vi "Test Plan - New Template (SubVI).vi"(8 "error in":errorcluster, 11 "Test Plan Name":string) -> (0 "error out":errorcluster, 2 "Give a name for new Test Plan 2":string, 3 "Test Type 2":T1 items=["Please Select", "Triaxial Shear", "Triaxial UU", "Shearbox", "Permeability", "Consolidation (Stepped Loading)/Swelling", "Saturation (Incremental)", "User Defined", "UCT", "Isotropic Consolidation"], 5 "save?":bool)   [LabVIEW 2019]
uses:
  Controls/Station - Test Type.ctl
  Controls/Test plan select-state.ctl
panel:
  in  "Test Type":u16(ring) items=["Please Select", "Triaxial Shear", "Triaxial UU", "Shearbox", "Permeability", "Consolidation (Stepped Loading)/Swelling", "Saturation (Incremental)", "User Defined", "UCT", "Isotropic Consolidation"]
  in  "OK":bool
  in  "Cancel":bool
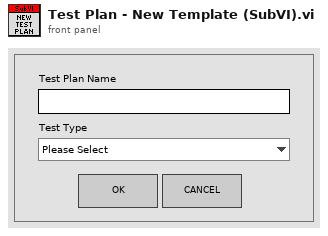
[diagram p1: front panel]
types:
  T1 = typedef "Station - Test Type.ctl" = u16
  T2 = enum16{"open", "replace", "create", "open or create", "replace or create", "replace or create with confirmation"}
  T3 = typedef "Test plan select-state.ctl" = enum16{"Init", "Idle", "Save", "Close"}
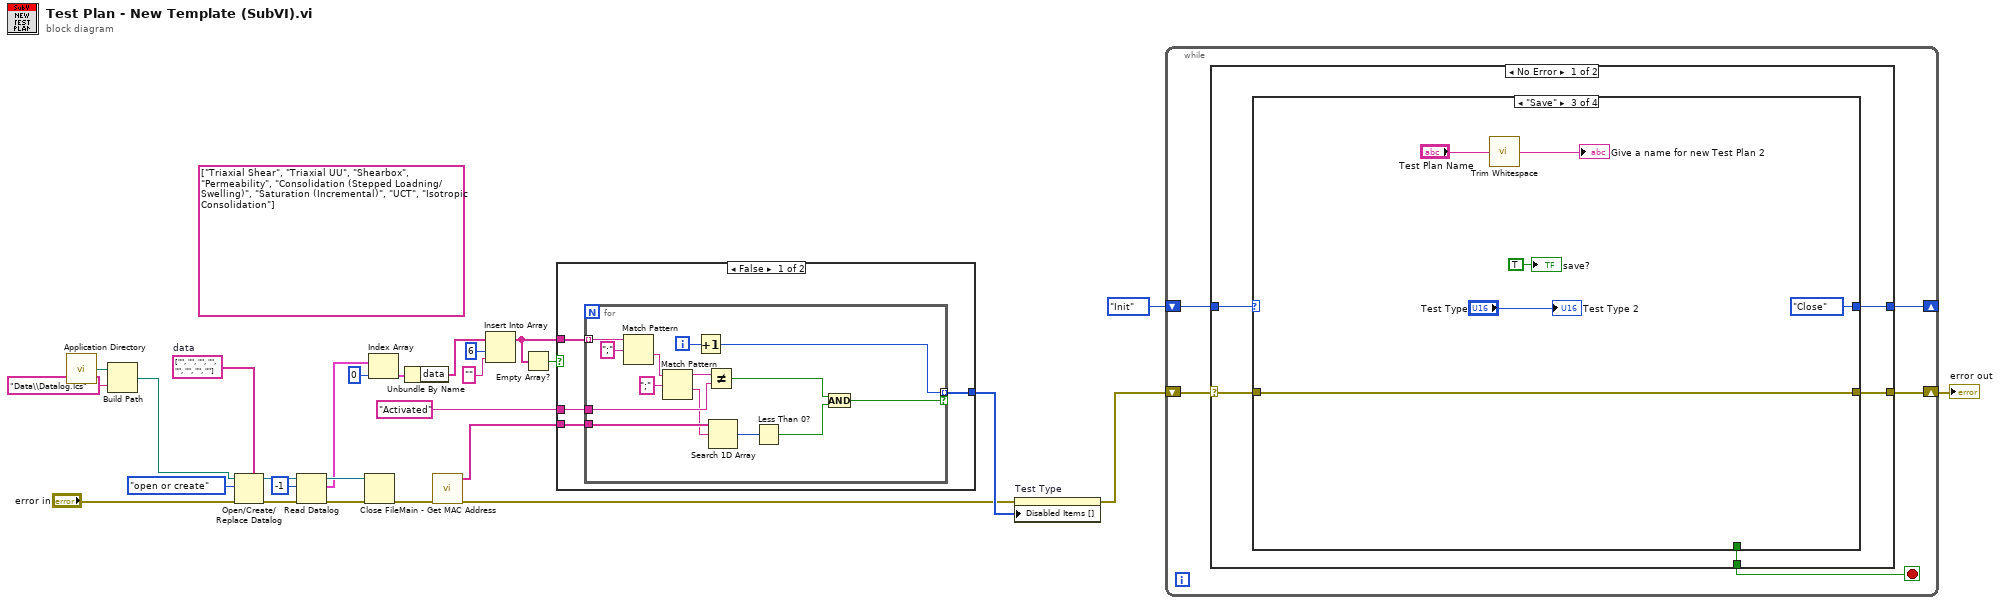
[diagram p0: block diagram]
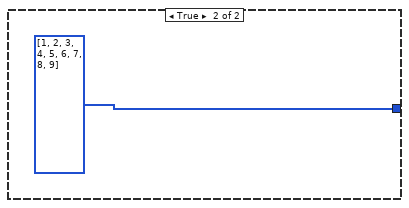
[diagram p2: hidden frame]
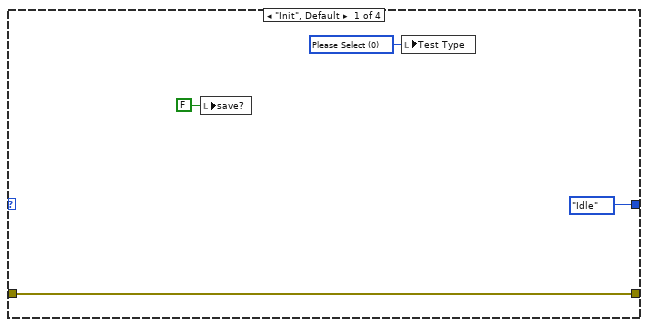
[diagram p3: hidden frame]
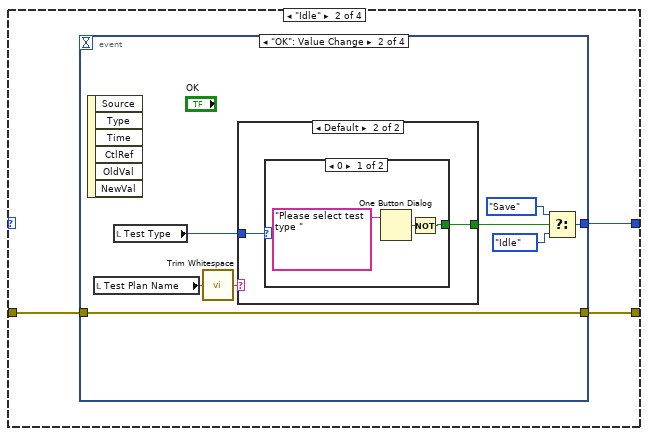
[diagram p4: hidden frame]
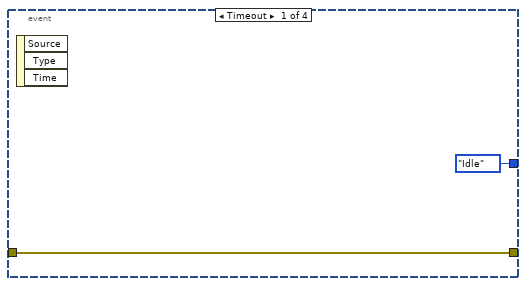
[diagram p5: hidden frame]
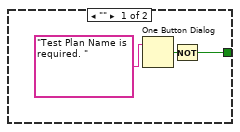
[diagram p6: hidden frame]
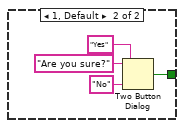
[diagram p7: hidden frame]
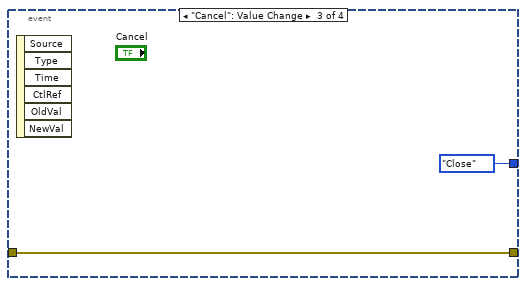
[diagram p8: hidden frame]
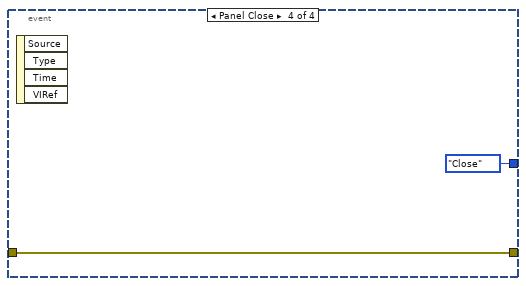
[diagram p9: hidden frame]
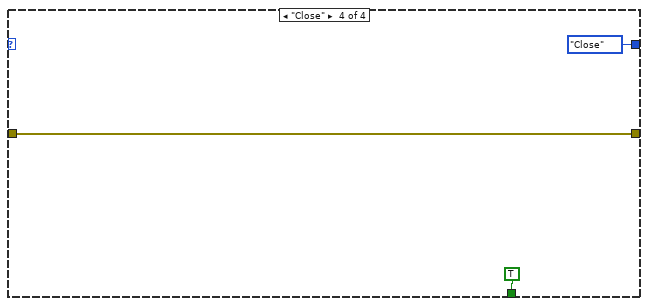
[diagram p10: hidden frame]
diagram:
  (unwired) string[] ["Triaxial Shear", "Triaxial UU", "Shearbox", "Permeability", "Consolidation (Stepped Loadning/Swelling)", "Saturation (Incremental)", "UCT", "Isotropic Consolidation"]
  w21 = string[] ["", "", "", "", "", "", "", ""]  # data
  n1 = call <vilib>:"Application Directory.vi"() -> ("Application Directory"=w25:path)
  n2 = Build Path(base path=w25, name or relative path="Data\\Datalog.lcs") -> (appended path=w13:path)
  n3 = Open/Create/Replace Datalog(5:w21, 8:"error in", 10:T2."open or create" ("operation (0:open)"), 11:w13) -> (0:w23:errorcluster, 3:w20:refnum<k1>)  [unwired: 2 in, 1 out]
  n4 = Read Datalog(4:w23, 6:-1 ("count (1)"), 7:w20) -> (0:w22:errorcluster, 2:w16:cluster{"data":string[]}[], 3:w19:refnum<k1>)
  n5 = Close File(refnum=w19, error in=w22) -> (error out=w5:errorcluster)  [unwired: 1 out]
  n6 = Index Array(array=w16, index=0) -> (element=w14:cluster{"data":string[]})
  n7 = Unbundle By Name(w14) -> ("data"=w10:string[])
  n8 = call "Main - Get MAC Address.vi"("error in (no error)"=w5) -> ("error out"=w4:errorcluster, "MAC Address"=w3:string[])  [unwired: 9 in]
  n9 = Insert Into Array(array=w10, index=6, new element="" ("new element/subarray")) -> (w7:string[])
  n10 = Empty Array?(array=w7) -> (empty?=w6:bool)
  n11 = case shown="False" w6 {
    tunnel: "Activated" -> [w31 _]
    tunnel: [w30 i32[] [1, 2, 3, 4, 5, 6, 7, 8, 9]] -> w11
    tunnel: w7 -> [w29 _]
    tunnel: w3 -> [w28 _]
    frame False {
      n12 = for {
        tunnel: w29 -> [w41] mode=indexing
        tunnel: w31 -> [w45]
        tunnel: [w43] -> w30 mode=indexing if=w32
        tunnel: w28 -> [w37]
        i -> [w44]
        n13 = Match Pattern(string=w41, regular expression=";") -> (after substring=w39:string)  [unwired: 1 in, 3 out]
        n14 = Match Pattern(string=w39, regular expression=";") -> (before substring=w38:string, after substring=w36:string)  [unwired: 1 in, 2 out]
        n15 = Increment(x=w44) -> (x+1=w43:i32)
        n16 = Not Equal?(x=w38, y=w45) -> (x != y?=w33:bool)
        n17 = Search 1D Array(1D array=w37, element=w36) -> (index of element=w35:i32)  [unwired: 1 in]
        n18 = Less Than 0?(x=w35) -> (x < 0?=w34:bool)
        n19 = And(x=w33, y=w34) -> (x .and. y?=w32:bool)
      }
    }
    frame True {
    }
  }
  n20 = property on="Test Type" class="Ring (strict)"(error in=w4, "Disabled Items []"=w11) -> (error out=w1:errorcluster)  [unwired: 1 in, 1 out]
  n21 = while {
    shift-right: [w50] -> w26
    shift-left: w1 -> [w51]
    shift-right: [w48] -> _
    shift-left: Test_plan_select-state."Init" -> [w49]
    stop <- w47 stop-if-true
    n22 = case shown="No Error" w51 {
      selector: w51 -> [w56 w99]
      tunnel: [w55 w99] -> w50
      tunnel: w49 -> [w54 _]
      tunnel: [w53 _] -> w48
      tunnel: [w52 _] -> w47
      frame No Error {
        n23 = case shown="\"Save\"" w54 {
          tunnel: w56 -> [w57 w63 w90 w98]
          tunnel: [w57 w62 w90 w98] -> w55
          tunnel: [Test_plan_select-state."Idle" w61 Test_plan_select-state."Close" Test_plan_select-state."Close"] -> w53
          tunnel: [_ _ _ TRUE] -> w52
          frame "Init", Default {
            w58 = T1 0 items=["Please Select", "Triaxial CU/CD Shear", "Triaxial UU", "UCT", "Shearbox", "Permeability", "CD Shearbox", "Consolidation", "1D Consolidation", "Saturation", "Swelling", "Custom"] ("Test Type")
            n24 = local write "save?"(FALSE ("save?")) -> ()
            n25 = local write "Test Type"(w58) -> ()
          }
          frame "Idle" {
            n26 = event shown="[1] \"OK\": Value Change" {
              selector: _ -> [_ _ _ _]
              dyn-events: _ -> [_ _ _ _]
              timeout: _ -> [_ _ _ _]
              tunnel: w63 -> [w65 w73 w86 w89]
              tunnel: [w65 w73 w86 w89] -> w62
              tunnel: [Test_plan_select-state."Idle" w70 Test_plan_select-state."Close" Test_plan_select-state."Close"] -> w61
              event Timeout {
                n27 = event-data() -> ()  [unwired: 1 in, 3 out]
              }
              event "OK": Value Change {
                n28 = event-data() -> ()  [unwired: 1 in, 6 out]
                n29 = local read "Test Plan Name"() -> (w67:string)
                n30 = local read "Test Type"() -> (w68:u16)
                n31 = call <vilib>:"Trim Whitespace.vi"("string"=w67) -> ("trimmed string"=w66:string)  [unwired: 1 in]
                n32 = case shown="Default" w66 {
                  tunnel: [w74 w78] -> w69
                  tunnel: w68 -> [_ w77]
                  frame "" {
                    n33 = One Button Dialog(message="Test Plan Name is required. ") -> (true=w76:bool)  [unwired: 1 in]
                    n34 = Not(x=w76) -> (.not. x?=w74:bool)
                  }
                  frame Default {
                    n35 = case shown="0" w77 {
                      tunnel: [w79 w82] -> w78
                      frame 0 {
                        n36 = One Button Dialog(message="Please select test type ") -> (true=w80:bool)  [unwired: 1 in]
                        n37 = Not(x=w80) -> (.not. x?=w79:bool)
                      }
                      frame 1, Default {
                        n38 = Two Button Dialog(message="Are you sure?", 1:"No" ("F button name (\"Cancel\")"), 2:"Yes" ("T button name (\"OK\")")) -> (T button?=w82:bool)
                      }
                    }
                  }
                }
                n39 = Select(t=Test_plan_select-state."Save", s=w69, f=Test_plan_select-state."Idle") -> (s? t:f=w70:T3)
              }
              event "Cancel": Value Change {
                n40 = event-data() -> ()  [unwired: 1 in, 6 out]
              }
              event Panel Close {
                n41 = event-data() -> ()  [unwired: 1 in, 4 out]
              }
            }
          }
          frame "Save" {
            n42 = call <vilib>:"Trim Whitespace.vi"("string"="Test Plan Name") -> ("trimmed string"=→"Give a name for new Test Plan 2":string)  [unwired: 1 in]
            "save?" <- TRUE ("save?")
            "Test Type 2" <- "Test Type"
          }
          frame "Close" {
          }
        }
      }
      frame Error {
      }
    }
  }
  "error out" <- w26
